vi "Spawn.vi"(9 "UID":string, 10 "Unified Actor":refnum<class "Actor.lvclass">, 11 "Core Actor in":refnum<class "Core Actor.lvclass">) -> (0 "Error out":errorcluster, 3 "Core Actor out":refnum<class "Core Actor.lvclass">)   [LabVIEW 2025, in "jettl.lvlib" / "Core Actor.lvlib" / "Core Actor.lvclass"]
uses:
  Core Actor.lvclass
  Actor/Actor.lvclass
  Attributes/Attributes/Attributes.lvclass
  Spawn.ctl
  Core Actor.lvclass/Core Actor.ctl
  Spawn/Spawn.lvlib
  jettl.lvlib
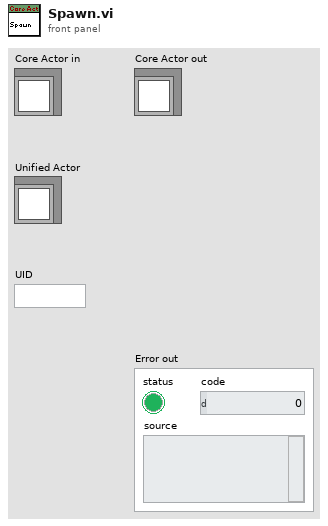
[diagram p1: front panel]
types:
  T1 = typedef "jettl.lvlib/Spawn.ctl" = cluster{"UID":string, "Parent Attributes":refnum<class "Attributes.lvclass">, "Queue of Self Attributes":refnum<queue>, "Queue of Error":refnum<queue>}
  T2 = typedef "jettl.lvlib/Core Actor.lvlib/Core Actor.lvclass/Child Attributes Map.ctl" = map{string, refnum<class "Attributes.lvclass">}
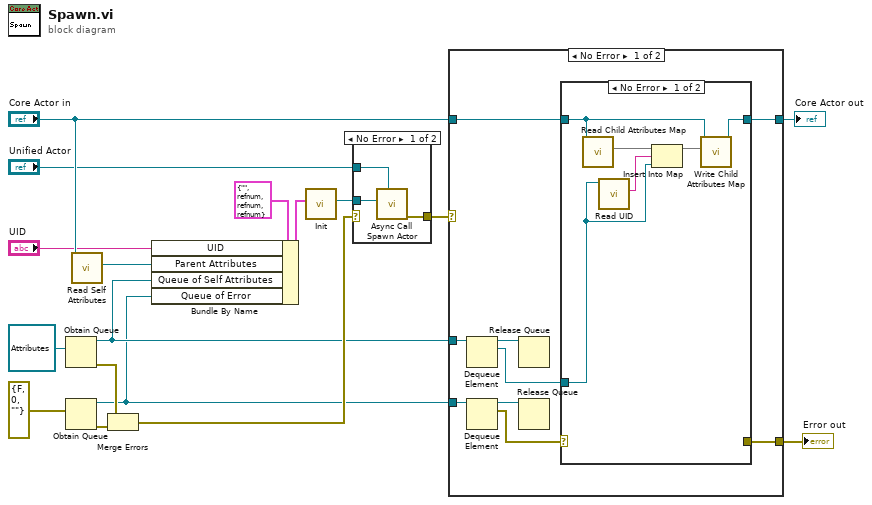
[diagram p0: block diagram]
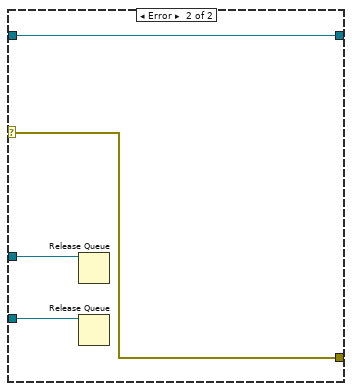
[diagram p4: hidden frame]
diagram:
  n1 = Obtain Queue(element data type=refnum<class "Attributes.lvclass"> refnum ("jettl.lvlib:Attributes.lvlib:Attributes.lvclass")) -> (queue out=w4:refnum<queue>, error out=w10:errorcluster)  [unwired: 4 in, 1 out]
  n2 = Obtain Queue(element data type=errorcluster {"status"=FALSE, "code"=0, "source"=""} ("Error")) -> (queue out=w3:refnum<queue>, error out=w9:errorcluster)  [unwired: 4 in, 1 out]
  n3 = call-dynamic "Read Self Attributes.vi"("Core Actor in"="Core Actor in") -> ("Self Attributes"=w6:refnum<class "Attributes.lvclass">)  [unwired: 10 in]
  n4 = Merge Errors(w10, w9) -> (w11:errorcluster)
  n5 = Bundle By Name(cluster=T1 {"UID"="", "Parent Attributes"=refnum, "Queue of Self Attributes"=refnum, "Queue of Error"=refnum} ("Config Actor"), "UID"="UID", "Parent Attributes"=w6, "Queue of Self Attributes"=w4, "Queue of Error"=w3) -> (w2:T1)
  n6 = call "Init.vi"("Spawn"=w2) -> ("Spawn"=w1:refnum<class "Spawn.lvclass">)  [unwired: 10 in]
  n7 = case shown="No Error" w11 {
    selector: w11 -> [_ w21]
    tunnel: [w18 w21] -> w14
    tunnel: "Unified Actor" -> [w20 _]
    tunnel: w1 -> [w19 _]
    frame No Error {
      n8 = call "Async Call Spawn Actor.vi"("Actor"=w20, "Spawn"=w19) -> ("Error out"=w18:errorcluster)  [unwired: 9 in]
    }
    frame Error {
    }
  }
  n9 = case shown="No Error" w14 {
    selector: w14 -> [_ w39]
    tunnel: "Core Actor in" -> [w30 w41]
    tunnel: [w29 w41] -> w17
    tunnel: w4 -> [w28 w42]
    tunnel: w3 -> [w26 w40]
    tunnel: [w22 w39] -> w15
    frame No Error {
      n10 = Dequeue Element(queue=w28) -> (queue out=w27:refnum<queue>, element=w24:refnum<class "Attributes.lvclass">)  [unwired: 2 in, 2 out]
      n11 = Dequeue Element(queue=w26) -> (queue out=w25:refnum<queue>, element=w23:errorcluster)  [unwired: 2 in, 2 out]
      n12 = Release Queue(queue=w27) -> ()  [unwired: 2 in, 3 out]
      n13 = Release Queue(queue=w25) -> ()  [unwired: 2 in, 3 out]
      n14 = case shown="No Error" w23 {
        selector: w23 -> [_ w37]
        tunnel: w30 -> [w34 w38]
        tunnel: [w33 w38] -> w29
        tunnel: w24 -> [w36 _]
        tunnel: [_ w37] -> w22
        frame No Error {
          n15 = call "Read Child Attributes Map.vi"("Core Actor in"=w34) -> ("Child Attributes Map"=w32:T2)  [unwired: 10 in]
          n16 = call-dynamic "Read UID.vi"("Attributes in"=w36) -> ("UID"=w35:string)  [unwired: 10 in]
          n17 = Insert Into Map(map in=w32, key=w35, value=w36) -> (map out=w31:T2)  [unwired: 2 out]
          n18 = call "Write Child Attributes Map.vi"("Child Attributes Map"=w31, "Core Actor in"=w34) -> ("Core Actor out"=w33:refnum<class "Core Actor.lvclass">)  [unwired: 9 in]
        }
        frame Error {
        }
      }
    }
    frame Error {
      n19 = Release Queue(queue=w42) -> ()  [unwired: 2 in, 3 out]
      n20 = Release Queue(queue=w40) -> ()  [unwired: 2 in, 3 out]
    }
  }
  "Core Actor out" <- w17
  "Error out" <- w15
